vi "Reset_Boric_Acid_Demineralized_Water_Mass_Flow_Integrator.vi"(0 "SI804.lvclass in":refnum<class "SI804.lvclass">, 2 "3 JSC31 FW421\nXA01":bool, 3 "3 JSC31 FW431\nXA01":bool, 5 "error in":errorcluster) -> (14 "SI804.lvclass out":refnum<class "SI804.lvclass">, 16 "Reset Boron Int":bool, 17 "Reset Demin Int":bool, 19 "error out":errorcluster)   [LabVIEW 2022 SP3, in "SI804.lvclass"]
uses:
  SI804.lvclass
  SI804.lvclass/SI804.ctl
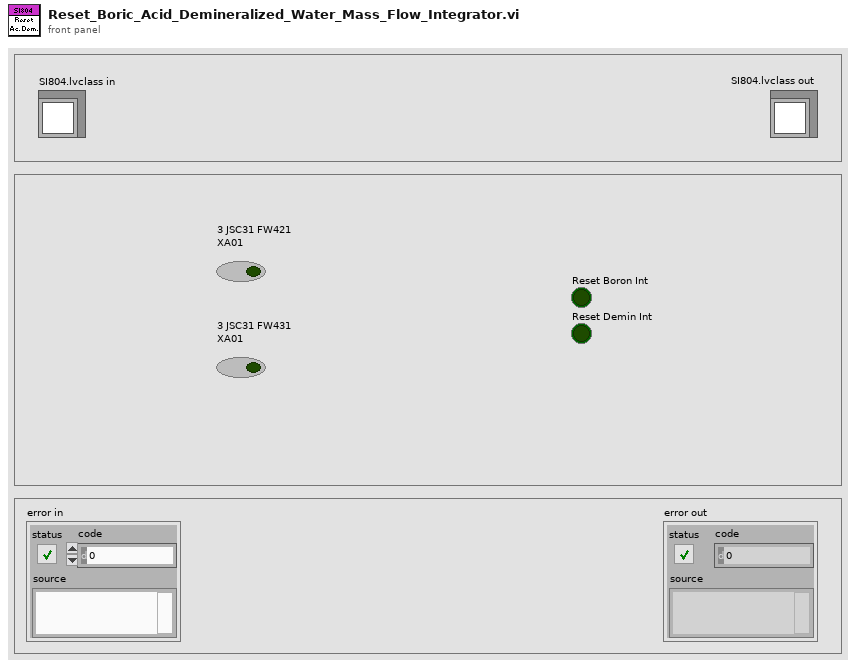
[diagram p1: front panel]
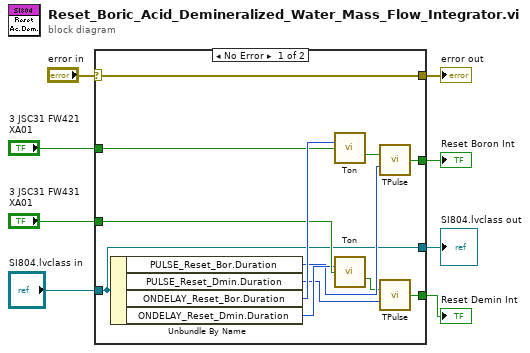
[diagram p0: block diagram]
diagram:
  n1 = case shown="No Error" "error in" {
    selector: "error in" -> [w10 w22]
    tunnel: "3 JSC31 FW421\nXA01" -> [w19 _]
    tunnel: "3 JSC31 FW431\nXA01" -> [w18 _]
    tunnel: "SI804.lvclass in" -> [w9 w21]
    tunnel: [w12 _] -> w4
    tunnel: [w11 _] -> w3
    tunnel: [w10 w22] -> w2
    tunnel: [w9 w21] -> w1
    frame No Error {
      n2 = Unbundle By Name(w9) -> ("PULSE_Reset_Bor.Duration"=w16:i32, "PULSE_Reset_Dmin.Duration"=w13:i32, "ONDELAY_Reset_Bor.Duration"=w20:i32, "ONDELAY_Reset_Dmin.Duration"=w17:i32)
      n3 = call "Ton.vi"("Ton"=w20, "input"=w19) -> ("Binary out"=w15:bool)  [unwired: 9 in, 4 out]
      n4 = call "Ton.vi"("Ton"=w17, "input"=w18) -> ("Binary out"=w14:bool)  [unwired: 9 in, 4 out]
      n5 = call "TPulse.vi"("trigger"=w15, "TPulse"=w16) -> ("output"=w12:bool)  [unwired: 11 in, 2 out]
      n6 = call "TPulse.vi"("trigger"=w14, "TPulse"=w13) -> ("output"=w11:bool)  [unwired: 11 in, 2 out]
    }
    frame Error {
    }
  }
  "Reset Boron Int" <- w4
  "Reset Demin Int" <- w3
  "error out" <- w2
  "SI804.lvclass out" <- w1
